vi "Read Configuration.vi"(8 "error in (no error)":errorcluster, 11 "Optical Power Meter in":refnum<class "Optical Power Meter.lvclass">) -> (0 "error out":errorcluster, 2 "Configuration":refnum<class "Configuration.lvclass">, 3 "Optical Power Meter out":refnum<class "Optical Power Meter.lvclass">)   [LabVIEW 2018, in "Optical Power Meter.lvlib" / "Optical Power Meter.lvclass"]
uses:
  Optical Power Meter.lvclass
  PPLs/Configuration/Configuration.lvlibp/Configuration.lvclass
  Optical Power Meter.lvclass/Optical Power Meter.ctl
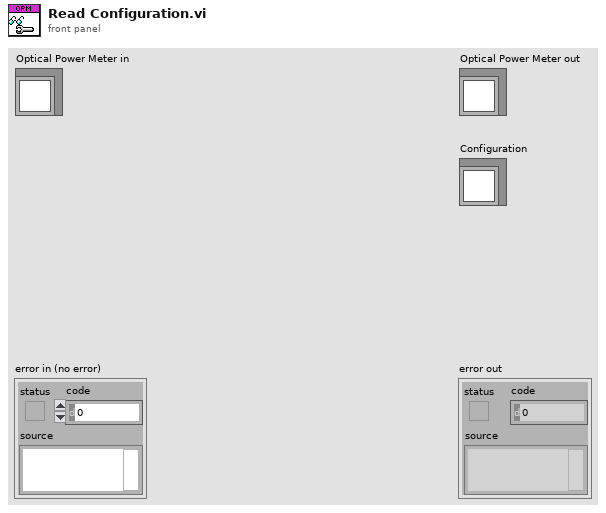
[diagram p1: front panel]
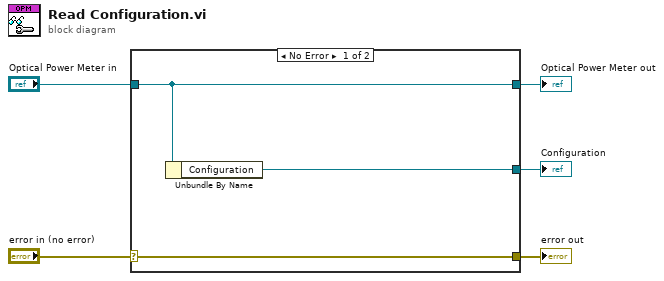
[diagram p0: block diagram]
diagram:
  n1 = case shown="No Error" "error in (no error)" {
    selector: "error in (no error)" -> [w8 w9]
    tunnel: [w8 w9] -> w4
    tunnel: [w7 w10] -> w2
    tunnel: "Optical Power Meter in" -> [w7 w10]
    tunnel: [w6 _] -> w1
    frame No Error {
      n2 = Unbundle By Name(w7) -> ("Configuration"=w6:refnum<class "Configuration.lvclass">)
    }
    frame Error {
    }
  }
  "error out" <- w4
  "Optical Power Meter out" <- w2
  "Configuration" <- w1
